vi "Init.vi"(8 "error in (no error)":errorcluster, 11 "Instrument Driver in":refnum<class "Instrument Driver.lvclass">) -> (0 "error out":errorcluster, 2 "Init Result":refnum<class "Acquired Result.lvclass">, 3 "Instrument Driver out":refnum<class "Instrument Driver.lvclass">)   [LabVIEW 2016, in "Instrument Driver.lvclass"]
uses:
  Instrument Driver.lvclass
  LabActor/Results/Acquired Result/Acquired Result.lvclass
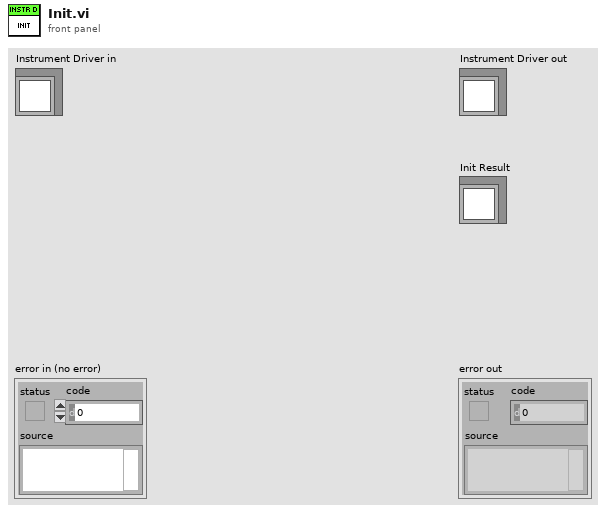
[diagram p1: front panel]
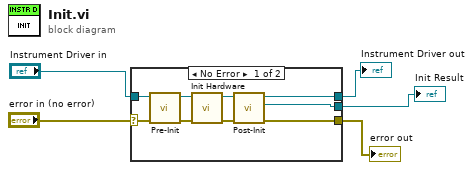
[diagram p0: block diagram]
diagram:
  n1 = case shown="No Error" "error in (no error)" {
    selector: "error in (no error)" -> [w8 w16]
    tunnel: [w7 w16] -> w4
    tunnel: [w9 w15] -> w2
    tunnel: "Instrument Driver in" -> [w10 w15]
    tunnel: [w6 _] -> w1
    frame No Error {
      n2 = call-dynamic "Pre-Init.vi"("error in (no error)"=w8, "Instrument Driver in"=w10) -> ("error out"=w12:errorcluster, "Instrument Driver out"=w14:refnum<class "Instrument Driver.lvclass">)  [unwired: 8 in]
      n3 = call-dynamic "Init Hardware.vi"("error in (no error)"=w12, "Instrument Driver in"=w14) -> ("error out"=w11:errorcluster, "Instrument Driver out"=w13:refnum<class "Instrument Driver.lvclass">)  [unwired: 8 in]
      n4 = call-dynamic "Post-Init.vi"("error in (no error)"=w11, "Instrument Driver in"=w13) -> ("error out"=w7:errorcluster, "Init Result"=w6:refnum<class "Acquired Result.lvclass">, "Instrument Driver out"=w9:refnum<class "Instrument Driver.lvclass">)  [unwired: 7 in]
    }
    frame Error {
    }
  }
  "error out" <- w4
  "Instrument Driver out" <- w2
  "Init Result" <- w1
